vi "Save2CSV.vi"(6 "Time Stamp?":bool=TRUE, 7 "File Name":string="ns_FLIM", 8 "error in":errorcluster, 9 "Data Name":string="Mix_Phase0", 10 "Data 2D Array":dbl[][](array[numeric]), 11 "Parent Directory":path) -> (0 "error out":errorcluster, 3 "save cancelled":bool)   [LabVIEW 2018]
uses:
  <vilib>/Utility/file.llb/Write Delimited Spreadsheet (DBL).vi
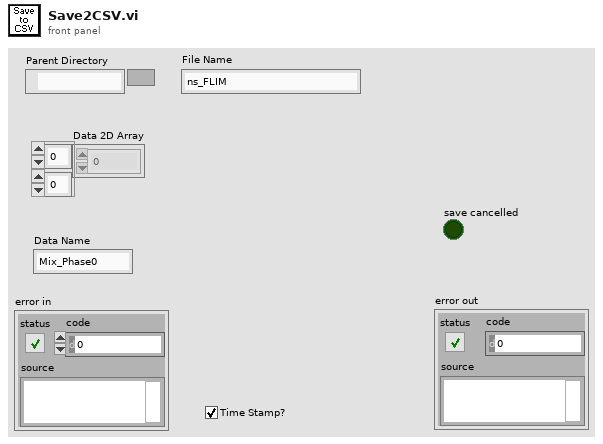
[diagram p1: front panel]
types:
  T1 = enum16{"open", "replace", "create", "open or create", "replace or create", "replace or create with confirmation"}
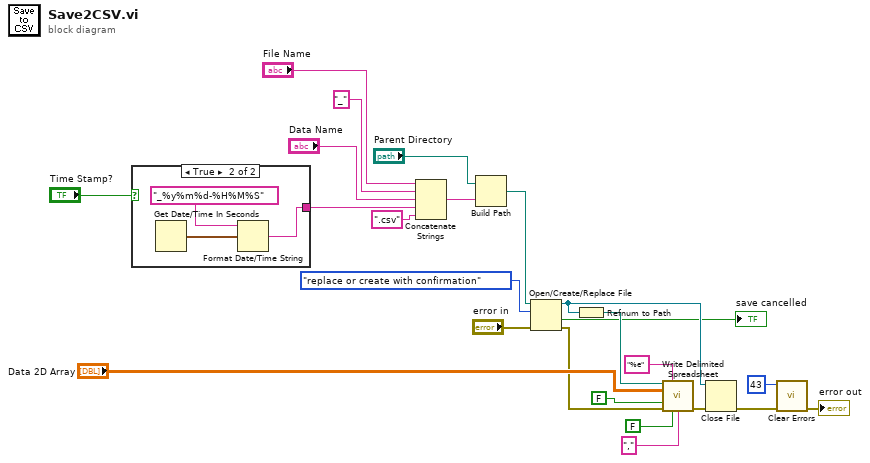
[diagram p0: block diagram]
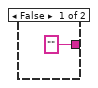
[diagram p2: hidden frame]
diagram:
  n1 = case shown="True" "Time Stamp?" {
    tunnel: ["" w26] -> w12
    frame False {
    }
    frame True {
      n2 = Get Date/Time In Seconds() -> (seconds since 1Jan1904=w27:timestamp)
      n3 = Format Date/Time String(time format string (%c)="_%y%m%d-%H%M%S", seconds (now)=w27) -> (date/time string=w26:string)  [unwired: 1 in]
    }
  }
  n4 = Concatenate Strings("File Name", "_" ("string"), "Data Name", w12, ".csv" ("string")) -> (w24:string)
  n5 = Build Path(base path="Parent Directory", name or relative path=w24) -> (appended path=w10:path)
  n6 = Open/Create/Replace File(file path (use dialog)=w10, error in="error in", operation (0:open)=T1."replace or create with confirmation") -> (refnum out=w2:refnum<file>, cancelled=→"save cancelled":bool, error out=w5:errorcluster)  [unwired: 3 in]
  n7 = Refnum to Path(1:w2) -> (0:w9:path)
  n8 = call-poly <vilib>:"Write Delimited Spreadsheet.vi"("file path (dialog if empty)"=w9, "format (%.3f)"="%e", "2D data"="Data 2D Array", "append to file? (new file:F)"=FALSE ("append to file? (F)"), "error in (no error)"=w5, "transpose? (no:F)"=FALSE ("transpose? (F)"), "delimiter (\\t)"="," ("delimiter (\\t)")) -> ("error out"=w4:errorcluster)  [unwired: 7 in, 1 out]
  n9 = Close File(refnum=w2, error in=w4) -> (error out=w3:errorcluster)  [unwired: 1 out]
  n10 = call <vilib>:"Clear Errors.vi"("error in (no error)"=w3, "specific error code to clear (0: all)"=43) -> ("error out"=→"error out":errorcluster)  [unwired: 4 in, 1 out]
